vi "Close.vi"(8 "error in (no error)":errorcluster caption="entrée d'erreur (pas d'erreur)", 11 "Process (Default) en entrée":refnum<class "Process (Default).lvclass">) -> (0 "error out":errorcluster caption="sortie d'erreur", 3 "Process (Default) en sortie":refnum<class "Process (Default).lvclass">)   [LabVIEW 2020, in "Library Instrument & Equipement.lvlib" / "Process (Default).lvclass"]
uses:
  Process (Default).lvclass
  Process (Default).lvclass/Process (Default).ctl
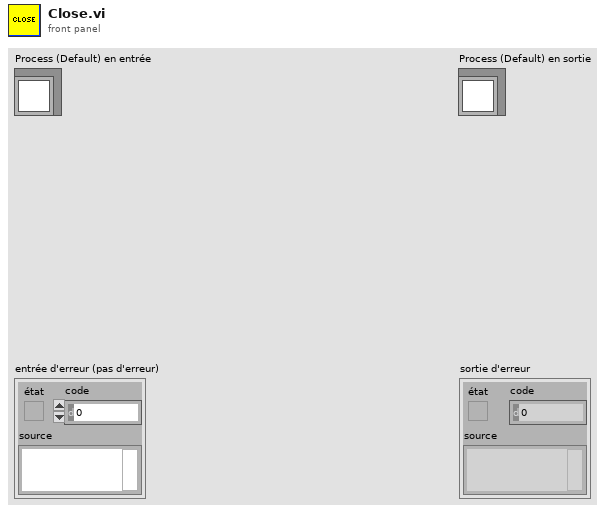
[diagram p1: front panel]
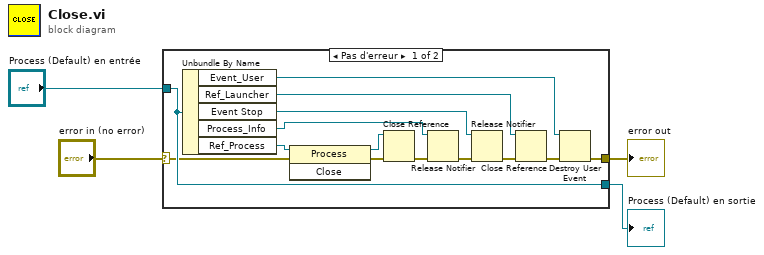
[diagram p0: block diagram]
diagram:
  n1 = case shown="Pas d'erreur" "error in (no error)" {
    selector: "error in (no error)" -> [w16 w20]
    tunnel: [w6 w20] -> w3
    tunnel: [w18 w19] -> w1
    tunnel: "Process (Default) en entrée" -> [w18 w19]
    frame No Error {
      n2 = Unbundle By Name(w18) -> ("Event_User"=w5:refnum<user-event>, "Ref_Launcher"=w9:refnum<vi>, "Event Stop"=w10:refnum<notifier>, "Process_Info"=w13:refnum<notifier>, "Ref_Process"=w17:refnum<k24>)
      n3 = invoke class="Process" method="Close"(reference=w17, error in=w16) -> (reference out=w14:refnum<k24>, error out=w15:errorcluster)  [unwired: 1 in, 1 out]
      n4 = Close Reference(reference=w14, error in (no error)=w15) -> (error out=w12:errorcluster)
      n5 = Release Notifier(notifier=w13, error in (no error)=w12) -> (error out=w11:errorcluster)  [unwired: 1 in, 2 out]
      n6 = Release Notifier(notifier=w10, error in (no error)=w11) -> (error out=w8:errorcluster)  [unwired: 1 in, 2 out]
      n7 = Close Reference(reference=w9, error in (no error)=w8) -> (error out=w7:errorcluster)
      n8 = Destroy User Event(user event=w5, error in=w7) -> (error out=w6:errorcluster)
    }
    frame Error {
    }
  }
  "error out" <- w3
  "Process (Default) en sortie" <- w1
